vi "TransferSegments.vi"(8 "segment number":i32, 10 "Channel (0)":u16 step=1, 11 "Handle Cluster":T1) -> (0 "Array":dbl[](array[numeric]), 2 "Data in Volts":dbl[][](array[numeric]))   [LabVIEW 2018]
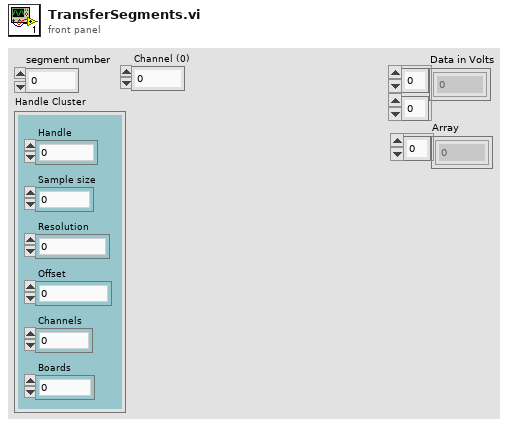
[diagram p1: front panel]
types:
  T1 = cluster{"Handle":u32, "Sample size":u32, "Resolution":i32, "Offset":i32, "Channels":u32, "Boards":u32}
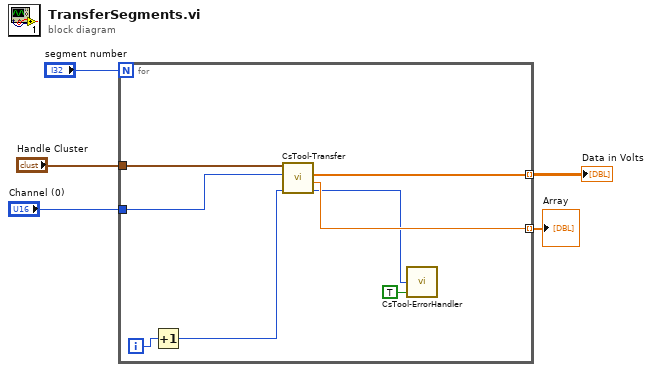
[diagram p0: block diagram]
diagram:
  n1 = for {
    N: "segment number" -> [_]
    tunnel: "Handle Cluster" -> [w13]
    tunnel: "Channel (0)" -> [w6]
    tunnel: [w12] -> w2 mode=indexing
    tunnel: [w11] -> w1 mode=indexing
    i -> [w8]
    n2 = Increment(x=w8) -> (x+1=w7:i32)
    n3 = call <userlib>:"CsTool-Transfer.vi"("Segment (1)"=w7, "Channel (0)"=w6, "Handle Cluster"=w13) -> ("Error Code"=w9:i32, "Actual Length"=w11:dbl, "Data in Volts"=w12:dbl[])  [unwired: 3 in, 1 out]
    n4 = call <userlib>:"CsTool-ErrorHandler.vi"("StopOnError (true)"=TRUE, "Error Code"=w9) -> ()  [unwired: 1 in, 1 out]
  }
  "Data in Volts" <- w2
  "Array" <- w1
